vi "Concatenar por Cursor.vi"(0 "WaveformGraph in":refnum<vi>, 1 "Cluster 3":T1, 2 "Flag":i32, 3 "Cursor 0":dbl, 4 "Cursor 1":dbl, 5 "error in":errorcluster) -> (15 "output cluster":T1, 19 "error out":errorcluster)   [LabVIEW 2020]
uses:
  TypeDef's/Dados consumidor.ctl
  <vilib>/Waveform/WDTOps.llb/WDT Waveform Duration DBL.vi
  <vilib>/Waveform/WDTOps.llb/WDT Get Waveform Subset DBL.vi
  <vilib>/Waveform/WDTOps.llb/WDT Append Waveforms DBL.vi
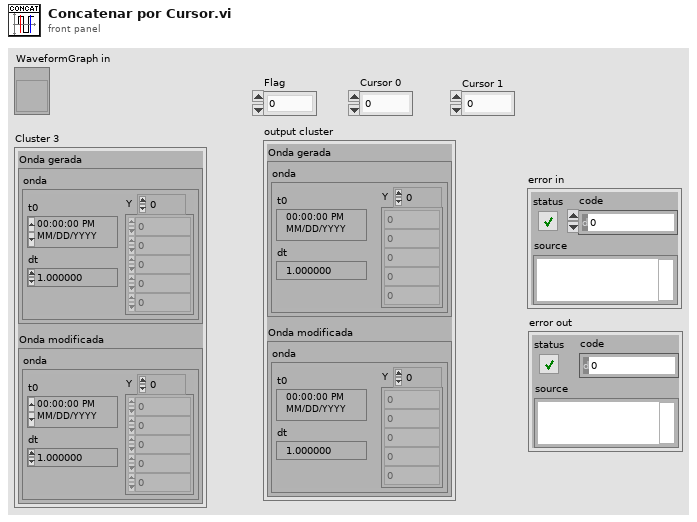
[diagram p1: front panel]
types:
  T1 = typedef "Dados consumidor.ctl" = cluster{"Onda gerada":cluster{"onda":waveform(dbl)}, "Onda modificada":cluster{"onda":waveform(dbl)}}
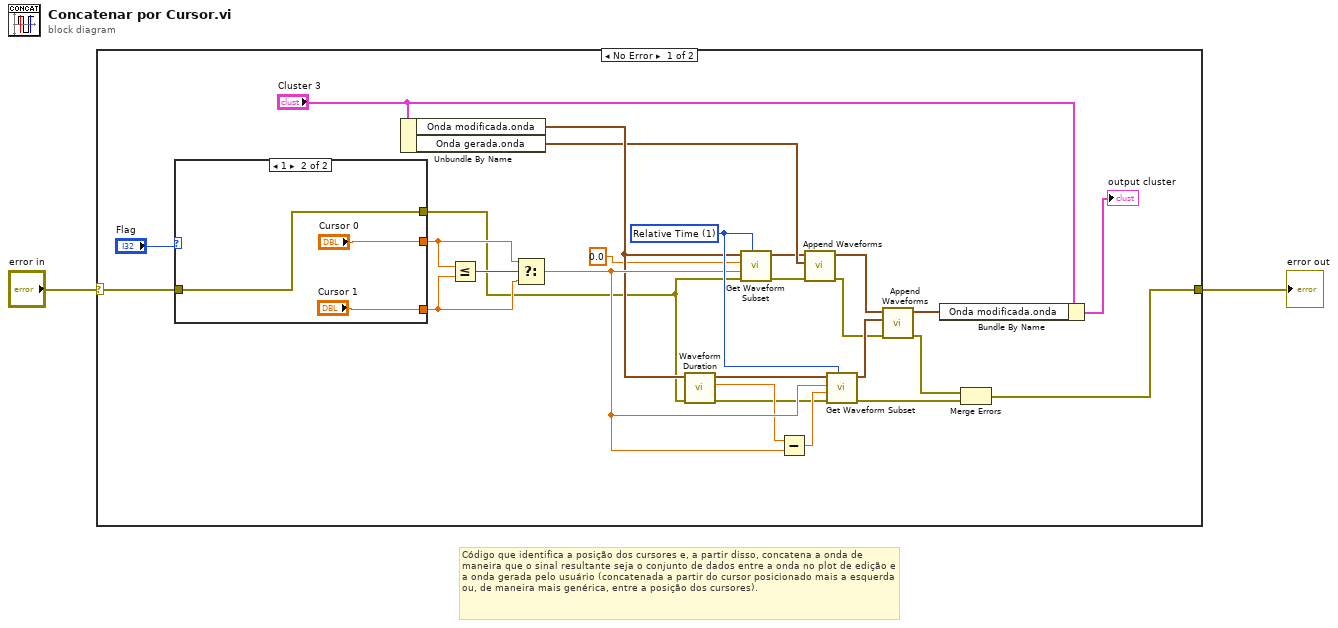
[diagram p0: block diagram]
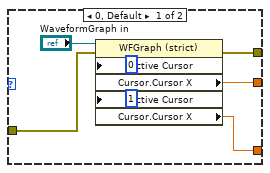
[diagram p2: hidden frame]
diagram:
  # "Código que identifica a posição dos cursores e, a partir disso, concatena a onda de maneira que o sinal resultante seja o conjunto de dados entre a onda no plot de edição e a onda gerada pelo usuário (concatenada a partir do cursor posicionado mais a esquerda ou, de maneira mais genérica, entre a posição dos cursores)."
  n1 = case shown="No Error" "error in" {
    selector: "error in" -> [w5 w39]
    tunnel: [w4 w39] -> w1
    frame No Error {
      w26 = u16 1 items=["Samples", "Relative Time"] ("start/duration format")
      n2 = case shown="1" "Flag" {
        tunnel: [w35 "Cursor 1"] -> w19
        tunnel: [w33 "Cursor 0"] -> w14
        tunnel: [w30 w36] -> w11
        tunnel: w5 -> [w29 w36]
        frame 0, Default {
          n3 = property on="Property Node" class="WFGraph (strict)"(reference="WaveformGraph in", error in=w29, "Active Cursor"=u32 0, "Active Cursor"=u32 1) -> (error out=w30:errorcluster, "Cursor.Cursor X"=w33:dbl, "Cursor.Cursor X"=w35:dbl)  [unwired: 1 out]
        }
        frame 1 {
        }
      }
      n4 = Unbundle By Name("Cluster 3") -> ("Onda modificada.onda"=w20:waveform(dbl), "Onda gerada.onda"=w18:waveform(dbl))
      n5 = Less Or Equal?(x=w14, y=w19) -> (x <= y?=w13:bool)
      n6 = Select(t=w14, s=w13, f=w19) -> (s? t:f=w24:dbl)
      n7 = call-poly <vilib>:"Waveform Duration.vi"("error in (no error)"=w11, "waveform in"=w20) -> ("error out"=w10:errorcluster, "duration"=w22:dbl, "waveform out"=w21:waveform(dbl))  [unwired: 7 in]
      n8 = call-poly <vilib>:"Get Waveform Subset.vi"("start/duration format"=w26, "error in (no error)"=w11, "duration"=w24, "start samples/time"=0.0, "waveform in"=w20) -> ("error out"=w9:errorcluster, "waveform out"=w16:waveform(dbl))  [unwired: 1 in, 2 out]
      n9 = Subtract(x=w22, y=w24) -> (x-y=w23:dbl)
      n10 = call-poly <vilib>:"Append Waveforms.vi"("error in (no error)"=w9, "waveform B"=w18, "waveform A"=w16) -> ("error out"=w8:errorcluster, "waveform out"=w17:waveform(dbl))  [unwired: 7 in]
      n11 = call-poly <vilib>:"Get Waveform Subset.vi"("start/duration format"=w26, "error in (no error)"=w10, "duration"=w23, "start samples/time"=w24, "waveform in"=w21) -> ("error out"=w6:errorcluster, "waveform out"=w25:waveform(dbl))  [unwired: 1 in, 2 out]
      n12 = call-poly <vilib>:"Append Waveforms.vi"("error in (no error)"=w8, "waveform B"=w25, "waveform A"=w17) -> ("error out"=w7:errorcluster, "waveform out"=w27:waveform(dbl))  [unwired: 7 in]
      n13 = Bundle By Name(cluster="Cluster 3", "Onda modificada.onda"=w27) -> (→"output cluster":T1)
      n14 = Merge Errors(w7, w6) -> (w4:errorcluster)
    }
    frame Error {
    }
  }
  "error out" <- w1
